vi "Set Message Data.vi"(6 "Data in":u8[](array[numeric]), 8 "error in (no error)":errorcluster, 9 "index":i32, 10 "Message Block Array in":u32[](array[numeric]), 11 "Udp Block Message Map in":map{i32, T1}(c390)) -> (0 "error out":errorcluster, 2 "Message Block Array out":u32[](array[numeric]), 3 "Udp Block Message Map out":map{i32, T1}(c390))   [LabVIEW 2020, in "UdpBlockMessage.lvlib"]
uses:
  UdpBlockMessage.lvlib
  ubm_value_type.ctl
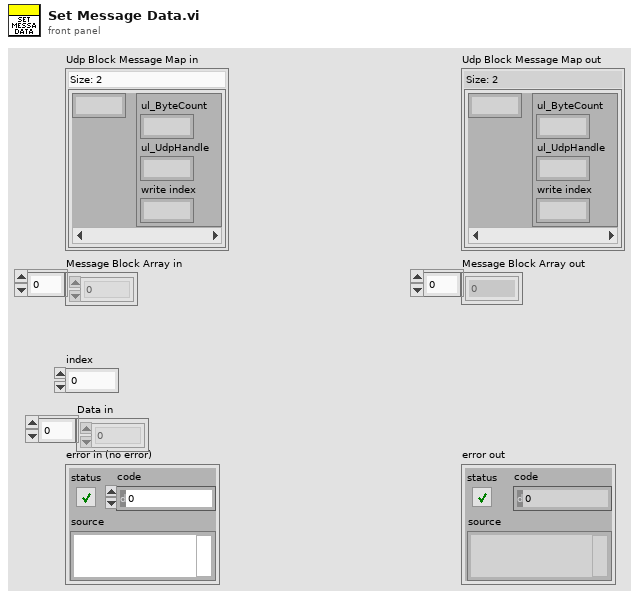
[diagram p1: front panel]
types:
  T1 = typedef "UdpBlockMessage.lvlib/ubm_value_type.ctl" = cluster{"ul_ByteCount":u32, "ul_UdpHandle":u32, "write index":u32}
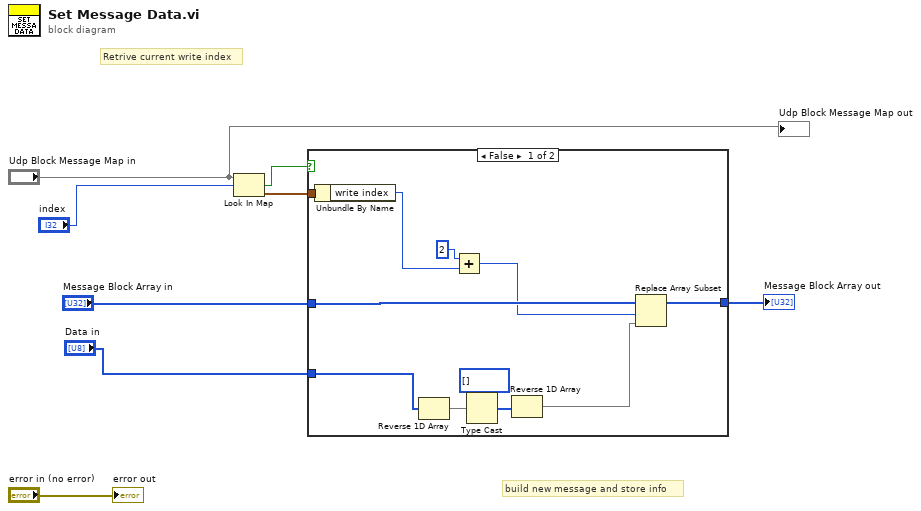
[diagram p0: block diagram]
diagram:
  # "build new message and store info"
  # "Retrive current write index"
  n1 = Look In Map(map="Udp Block Message Map in", key="index") -> (key not found?=w1:bool, value=w3:T1)  [unwired: 1 in]
  n2 = case shown="False" w1 {
    tunnel: "Message Block Array in" -> [w19 w20]
    tunnel: [w18 w20] -> w7
    tunnel: w3 -> [w16 _]
    tunnel: "Data in" -> [w10 _]
    frame False {
      n3 = Unbundle By Name(w16) -> ("write index"=w15:u32)
      n4 = Reverse 1D Array(array=w10) -> (reversed array=w13:u8[])
      n5 = Add(x=u32 2, y=w15) -> (x+y=w14:u32)
      n6 = Type Cast(type=u32[] [] ("Buf"), x=w13) -> (*(type *) &x=w12:u32[])
      n7 = Reverse 1D Array(array=w12) -> (reversed array=w9:u32[])
      n8 = Replace Array Subset(array=w19, new element=w9, index=w14) -> (w18:u32[])
    }
    frame True {
    }
  }
  "Message Block Array out" <- w7
  "error out" <- "error in (no error)"
  "Udp Block Message Map out" <- "Udp Block Message Map in"
